vi "MICSD Abort.vi"(8 "error in (no error)":errorcluster, 11 "VISA Resource Name":refnum<visa-resource-name>) -> (0 "error out":errorcluster, 3 "dup VISA Resource Name":refnum<visa-resource-name>)   [LabVIEW 2020]
uses:
  <vilib>/Instr/_visa.llb/VISA Configure Serial Port (Instr).vi
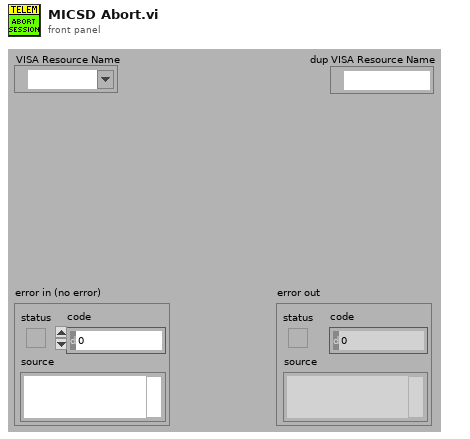
[diagram p1: front panel]
types:
  T1 = cluster{"Command Token":u8, "Length":u16, "Pack Data":u8[]}
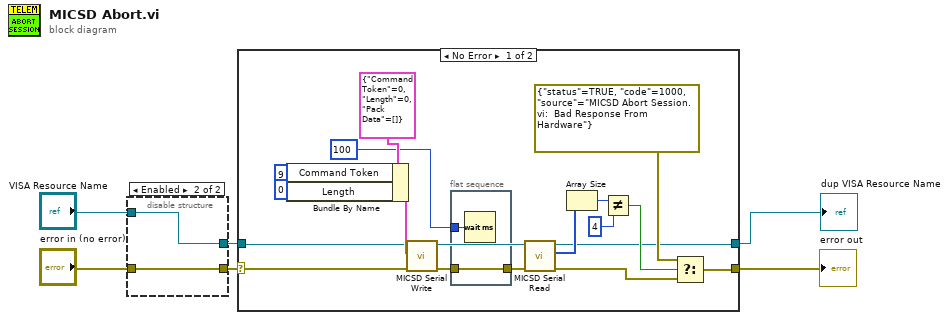
[diagram p0: block diagram]
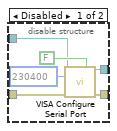
[diagram p2: hidden frame]
diagram:
  n1 = disable-structure shown="Enabled" {
    disable-tunnel: [w10 w13] -> w6
    disable-tunnel: [w9 w14] -> w5
    disable-tunnel: "VISA Resource Name" -> [w8 w14]
    disable-tunnel: "error in (no error)" -> [w7 w13]
    frame Disabled {
      n2 = call-poly "VISA Configure Serial Port"("VISA resource name"=w8, "Enable Termination\nChar (T)"=FALSE ("Enable Termination\nChar (T)"), "baud rate (9600)"=u32 230400, "error in (no error)"=w7) -> ("VISA resource name out"=w9:refnum<visa-resource-name>, "error out"=w10:errorcluster)  [unwired: 10 in]
    }
    frame Enabled {
    }
  }
  n3 = case shown="No Error" w6 {
    selector: w6 -> [w23 w36]
    tunnel: [w32 w36] -> w1
    tunnel: w5 -> [w21 w35]
    tunnel: [w16 w35] -> w2
    frame No Error {
      n4 = Bundle By Name(cluster=T1 {"Command Token"=0, "Length"=0, "Pack Data"=[]} ("Write Data"), "Command Token"=u8 9, "Length"=u16 0) -> (w29:T1)
      n5 = call "MICSD Serial Write.vi"("error in (no error)"=w23, "Write Data"=w29, "VISA Resource Name"=w21) -> ("error out"=w30:errorcluster, "DUP Visa Resource Name"=w26:refnum<visa-resource-name>)  [unwired: 7 in]
      n6 = flat-sequence {
        tunnel: w30 -> [w34]
        tunnel: [w34] -> w27
        tunnel: u16 100 ("x") -> [w33]
        frame #0 {
          n7 = Wait (ms)(milliseconds to wait=w33) -> ()  [unwired: 1 out]
        }
      }
      n8 = call "MICSD Serial Read.vi"("error in (no error)"=w27, "VISA Resource Name"=w26) -> ("error out"=w22:errorcluster, "Read Data"=w20:u8[], "DUP Visa Resource Name"=w16:refnum<visa-resource-name>)  [unwired: 7 in]
      n9 = Array Size(array=w20) -> (size(s)=w19:i32)
      n10 = Not Equal?(x=w19, y=4) -> (x != y?=w18:bool)
      n11 = Select(t=errorcluster {"status"=TRUE, "code"=1000, "source"="MICSD Abort Session.vi:  Bad Response From Hardware"} ("error IO"), s=w18, f=w22) -> (s? t:f=w32:errorcluster)
    }
    frame Error {
    }
  }
  "dup VISA Resource Name" <- w2
  "error out" <- w1
